vi "MakePythonArgumentList.vi"(1 "Arg 6":string, 2 "Arg 5":string, 3 "Arg 4":string, 4 "Arg 3":string, 5 "Arg 2":string, 6 "Arg 1":string) -> (0 "Args Out":string)   [LabVIEW 2014]
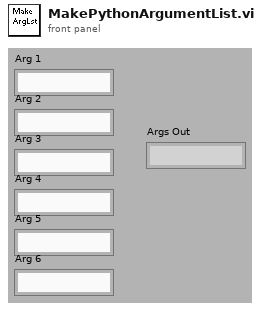
[diagram p1: front panel]
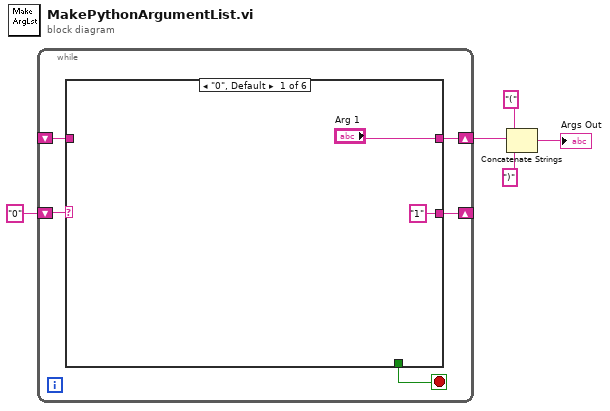
[diagram p0: block diagram]
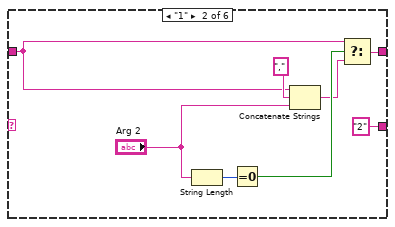
[diagram p2: hidden frame]
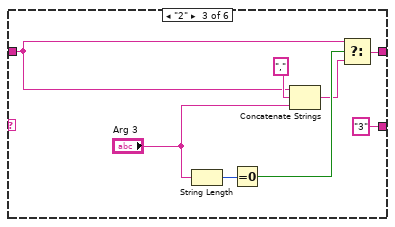
[diagram p3: hidden frame]
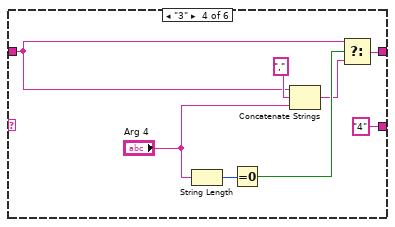
[diagram p4: hidden frame]
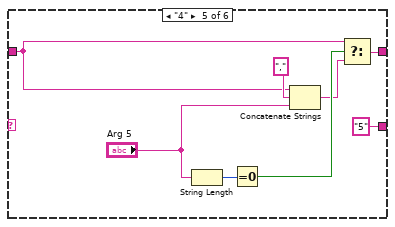
[diagram p5: hidden frame]
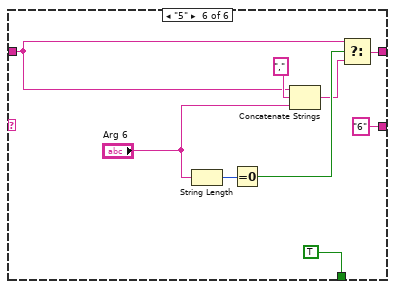
[diagram p6: hidden frame]
diagram:
  n1 = while {
    shift-right: [w6] -> _
    shift-left: "0" -> [w10]
    shift-right: [w9] -> w1
    shift-left: _ -> [w7]
    stop <- w8 stop-if-true
    n2 = case shown="\"0\", Default" w10 {
      tunnel: ["Arg 1" w16 w24 w32 w40 w49] -> w9
      tunnel: [_ _ _ _ _ TRUE] -> w8
      tunnel: w7 -> [_ w14 w22 w30 w38 w47]
      tunnel: ["1" "2" "3" "4" "5" "6"] -> w6
      frame "0", Default {
      }
      frame "1" {
        n3 = String Length(string="Arg 2") -> (length=w19:i32)
        n4 = Equal To 0?(x=w19) -> (x = 0?=w20:bool)
        n5 = Concatenate Strings(w14, ",", "Arg 2") -> (w15:string)
        n6 = Select(t=w14, s=w20, f=w15) -> (s? t:f=w16:string)
      }
      frame "2" {
        n7 = String Length(string="Arg 3") -> (length=w27:i32)
        n8 = Equal To 0?(x=w27) -> (x = 0?=w28:bool)
        n9 = Concatenate Strings(w22, ",", "Arg 3") -> (w23:string)
        n10 = Select(t=w22, s=w28, f=w23) -> (s? t:f=w24:string)
      }
      frame "3" {
        n11 = String Length(string="Arg 4") -> (length=w35:i32)
        n12 = Equal To 0?(x=w35) -> (x = 0?=w36:bool)
        n13 = Concatenate Strings(w30, ",", "Arg 4") -> (w31:string)
        n14 = Select(t=w30, s=w36, f=w31) -> (s? t:f=w32:string)
      }
      frame "4" {
        n15 = String Length(string="Arg 5") -> (length=w43:i32)
        n16 = Equal To 0?(x=w43) -> (x = 0?=w44:bool)
        n17 = Concatenate Strings(w38, ",", "Arg 5") -> (w39:string)
        n18 = Select(t=w38, s=w44, f=w39) -> (s? t:f=w40:string)
      }
      frame "5" {
        n19 = String Length(string="Arg 6") -> (length=w52:i32)
        n20 = Equal To 0?(x=w52) -> (x = 0?=w53:bool)
        n21 = Concatenate Strings(w47, ",", "Arg 6") -> (w48:string)
        n22 = Select(t=w47, s=w53, f=w48) -> (s? t:f=w49:string)
      }
    }
  }
  n23 = Concatenate Strings("(", w1, ")") -> (→"Args Out":string)
